vi "BasicControlPathAndTypeInSubPanel_Tests.vi"(11 "error in":errorcluster) -> (15 "error out":errorcluster)   [LabVIEW 2016, in "DronaTest.lvlib"]
uses:
  DronaTest.lvlib
  APIs/Stimulus/ControlValue/ValueSignalByPathString.vi
  APIs/Assert/AssertControlValue/Equal.vi
  <vilib>/addons/_JKI Toolkits/Caraya/classes/Test/Test.lvclass
  Drona.lvlib
  APIs/Stimulus/ControlValue/ControlValue.lvlib
  APIs/Assert/AssertControlValue/AssertControlValue.lvlib
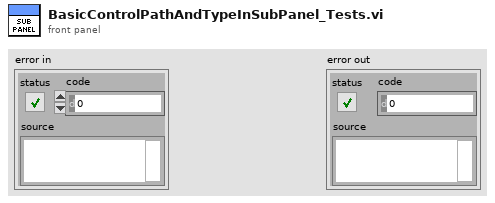
[diagram p1: front panel]
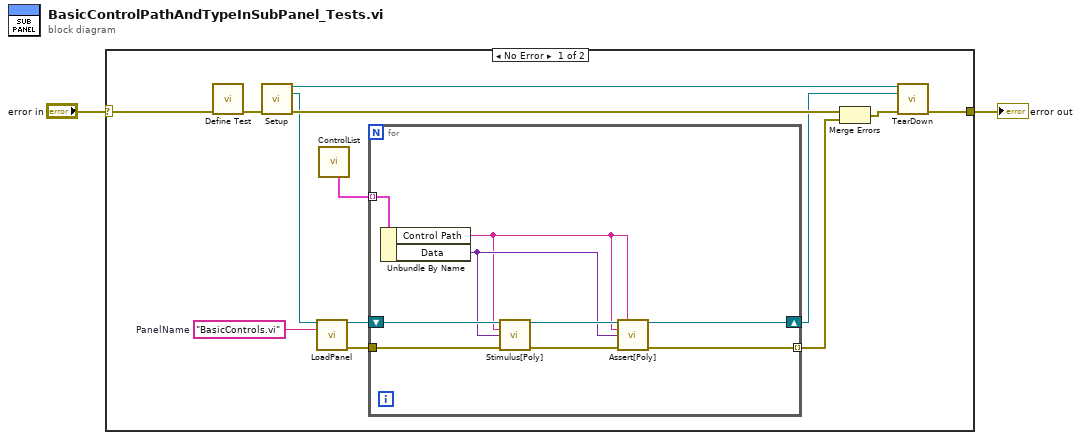
[diagram p0: block diagram]
diagram:
  n1 = case shown="No Error" "error in" {
    selector: "error in" -> [w14 w25]
    tunnel: [w6 w25] -> w1
    frame No Error {
      w10 = "BasicControls.vi"  # PanelName
      n2 = call <vilib>:"Define Test.vi"("error in (no error)"=w14) -> ("error out"=w12:errorcluster)  [unwired: 9 in, 1 out]
      n3 = call "Setup.vi"("error in (no error)"=w12) -> ("Application Ref"=w5:refnum<vi>, "VI out"=w4:refnum<vi>, "error out"=w7:errorcluster)  [unwired: 12 in]
      n4 = call "LoadPanel.vi"("VI in"=w4, "Item Name"=w10) -> ("VI out"=w9:refnum<vi>, "error out"=w8:errorcluster)  [unwired: 12 in]
      n5 = call "ControlList.vi"() -> ("SubPanel"=w11:cluster{"Control Path":string, "Data":variant}[])  [unwired: 6 in, 5 out]
      n6 = for {
        shift-right: [w24] -> w3
        shift-left: w9 -> [w20]
        tunnel: [w17] -> w15 mode=indexing
        tunnel: w11 -> [w21] mode=indexing
        tunnel: w8 -> [w16]
        n7 = Unbundle By Name(w21) -> ("Control Path"=w18:string, "Data"=w19:variant)
        n8 = call-poly "Stimulus[Poly].vi"("VI Reference In"=w20, "Control Path"=w18, "Value (Signaling)"=w19, "error in"=w16) -> ("VI Reference Out"=w22:refnum<vi>, "error out"=w23:errorcluster)  [unwired: 10 in]
        n9 = call-poly "Assert[Poly].vi"("VI Reference In"=w22, "Test Label"=w18, "Control Path"=w18, "Control Value"=w19, "Error In"=w23) -> ("VI Reference Out"=w24:refnum<vi>, "Error Out"=w17:errorcluster)  [unwired: 8 in, 1 out]
      }
      n10 = Merge Errors(w7, w15) -> (w13:errorcluster)
      n11 = call "TearDown.vi"("Application Ref"=w5, "VI in"=w3, "error in (no error)"=w13) -> ("error out"=w6:errorcluster)  [unwired: 12 in]
    }
    frame Error {
    }
  }
  "error out" <- w1
